vi "ZMQ_slave_Create.vi"(8 "error in (no error)":errorcluster, 10 "endpoint":string="tcp://127.0.0.1:5555", 11 "reference in":refnum<class "ZMQ_slave.lvclass">) -> (0 "error out":errorcluster, 3 "reference out":refnum<class "ZMQ_slave.lvclass">)   [LabVIEW 2019, in "CommandResponse communication.lvlib" / "ZMQ_slave.lvclass"]
doc: "Constructor."
uses:
  ZMQ_slave.lvclass
  C:/Program Files/National Instruments/LabVIEW 2019/vi.lib/addons/_AddQ/G#Object/G#Object.lvclass
  C:/Barkhausen mmWave radar/Development/LV/Barkhausen mmWave hardware control/Host/Intertarget communication/CR slave_class/CR slave.lvclass
  <vilib>/addons/zeromq/socket_type.ctl
  <vilib>/addons/_AddQ/G#Object/G#Object.lvclass
  CR slave_class/CR slave.lvclass
  <vilib>/addons/zeromq/zmq_context.lvclass
  <vilib>/addons/zeromq/zmq_socket.lvclass
  <vilib>/addons/zeromq/zeromq.lvlib
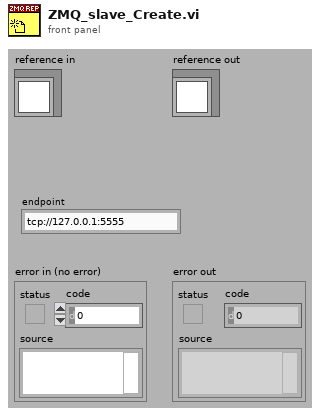
[diagram p1: front panel]
types:
  T1 = typedef "zeromq.lvlib/socket_type.ctl" = enum8{"ZMQ_PAIR", "ZMQ_PUB", "ZMQ_SUB", "ZMQ_REQ", "ZMQ_REP", "ZMQ_DEALER", "ZMQ_ROUTER", "ZMQ_PULL", "ZMQ_PUSH", "ZMQ_XPUB", "ZMQ_XSUB"}
  T2 = typedef "CommandResponse communication.lvlib/ZMQ_slave.lvclass/ObjectAttributesRef.ctl" = refnum<data-value>
  T3 = typedef "CommandResponse communication.lvlib/ZMQ_slave.lvclass/ObjectAttributes.ctl" = cluster{"ZMQ context":refnum<class "zmq_context.lvclass">, "ZMQ socket":refnum<class "zmq_socket.lvclass">, "endpoint":string}
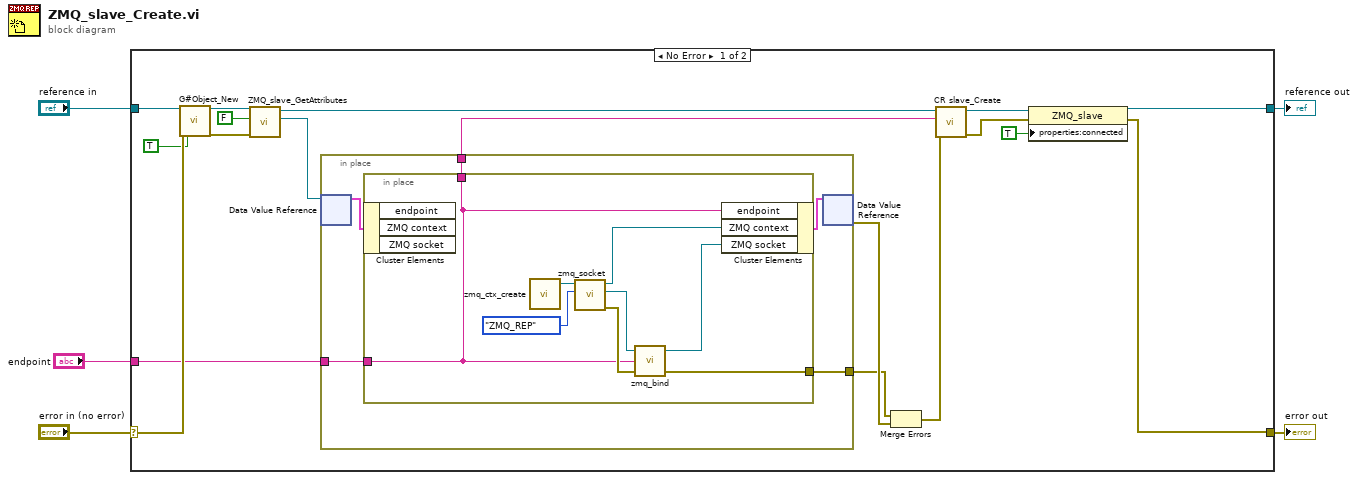
[diagram p0: block diagram]
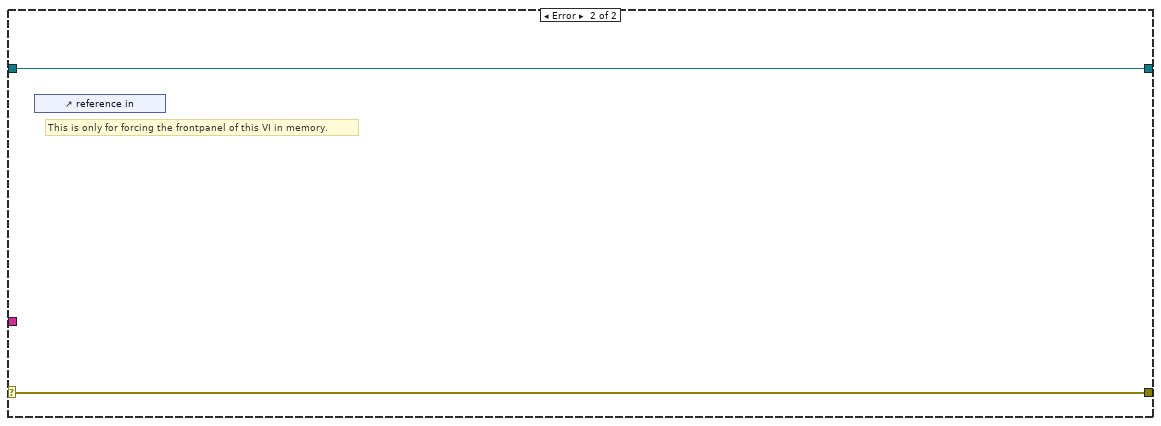
[diagram p2: hidden frame]
diagram:
  n1 = case shown="No Error" "error in (no error)" {
    selector: "error in (no error)" -> [w22 w38]
    tunnel: [w7 w38] -> w4
    tunnel: [w6 w37] -> w2
    tunnel: "reference in" -> [w23 w37]
    tunnel: "endpoint" -> [w12 _]
    frame No Error {
      n2 = call <vilib>:"G#Object_New.vi"("reference in"=w23, "error in (no error)"=w22, "user counter (T)?"=TRUE ("User Counter")) -> ("reference out"=w17:refnum<class "ZMQ_slave.lvclass">, "error out"=w16:errorcluster)  [unwired: 14 in, 1 out]
      n3 = call "ZMQ_slave_GetAttributes.vi"("error in (no error)"=w16, "return data? (T)"=FALSE ("return data"), "reference in"=w17) -> ("attributes ref"=w19:T2, "reference out"=w15:refnum<class "ZMQ_slave.lvclass">)  [unwired: 5 in, 2 out]
      n4 = in-place {
        in-place-border: [w26] -> w13
        in-place-border: w12 -> [w25]
        in-place-border: [w24] -> w11
        n5 = in-place-dvr #1(w19) -> (w27:T3)  [unwired: 1 out]
        n6 = in-place {
          in-place-border: [w32] -> w26
          in-place-border: w25 -> [w32]
          in-place-border: [w31] -> w24
          n7 = in-place-cluster #2(w27) -> ()  [unwired: 3 out]
          n8 = call <vilib>:"zmq_ctx_create.vi"() -> ("context out"=w34:refnum<class "zmq_context.lvclass">)  [unwired: 4 in, 1 out]
          n9 = call <vilib>:"zmq_socket.vi"("socket type"=socket_type."ZMQ_REP", "context in"=w34) -> ("error out"=w36:errorcluster, "socket out"=w33:refnum<class "zmq_socket.lvclass">, "context out"=w30:refnum<class "zmq_context.lvclass">)  [unwired: 3 in]
          n10 = call <vilib>:"zmq_bind.vi"("error in"=w36, "endpoint"=w32, "socket in"=w33) -> ("error out"=w31:errorcluster, "socket out"=w29:refnum<class "zmq_socket.lvclass">)  [unwired: 1 in]
          n11 = in-place-cluster #2("endpoint"=w32, "ZMQ context"=w30, "ZMQ socket"=w29) -> (w28:T3)
        }
        n12 = in-place-dvr #1(w28) -> (w20:errorcluster)  [unwired: 1 out]
      }
      n13 = Merge Errors(w11, w20) -> (w14:errorcluster)
      n14 = call "CR slave_Create.vi"("error in (no error)"=w14, "ID"=w13, "reference in"=w15) -> ("error out"=w8:errorcluster, "reference out"=w10:refnum<class "ZMQ_slave.lvclass">)  [unwired: 7 in]
      n15 = property class="ZMQ_slave"(reference=w10, error in=w8, "properties:connected"=TRUE) -> (reference out=w6:refnum<class "ZMQ_slave.lvclass">, error out=w7:errorcluster)
    }
    frame Error {
      # "This is only for forcing the frontpanel of this VI in memory."
      n16 = control-ref of="reference in"() -> ()  [unwired: 1 out]
    }
  }
  "error out" <- w4
  "reference out" <- w2
